vi "TLTSPB_Example.vi"() -> ()   [LabVIEW 2023]
uses:
  Program Files/National Instruments/LabVIEW 2020/instr.lib/TLTSP/TLTSP.llb/z_StateMachineVorlageV2011.ctl
panel:
  out "XY Graph":T1(graph)
  out "Humidity":dbl
  out "Temperature":dbl caption="Temperature Ch1"
  in  "Stop":bool
  in  "Start":bool
  in  "Quit":bool
  in  "Tab Control":enum32{"Page 1", "Page 2"}(tab)
  in  "error in":errorcluster
  out "error out":errorcluster
  in  "Handle":refnum<visa-resource-name>
  in  "State210":T2 caption="States"
  out "State100":T2 caption="States"
  out "user event out":refnum<user-event>
  out "Connected":bool
  out "UserEventRefNum":refnum<event-registration>
  out "Temperature 2":dbl[](array[numeric])
  out "Humidity 2":dbl[](array[numeric])
  out "Time":timestamp[](array[timestamp])
  in  "Delay [ms]":u32=50
  out "Serial Number":string
  out "Device Name":string
  out "Manufacturer Name":string
  out "Firmware Revision":string
  out "Statuszeile":string
  # "Thorlabs TSP01B Example"
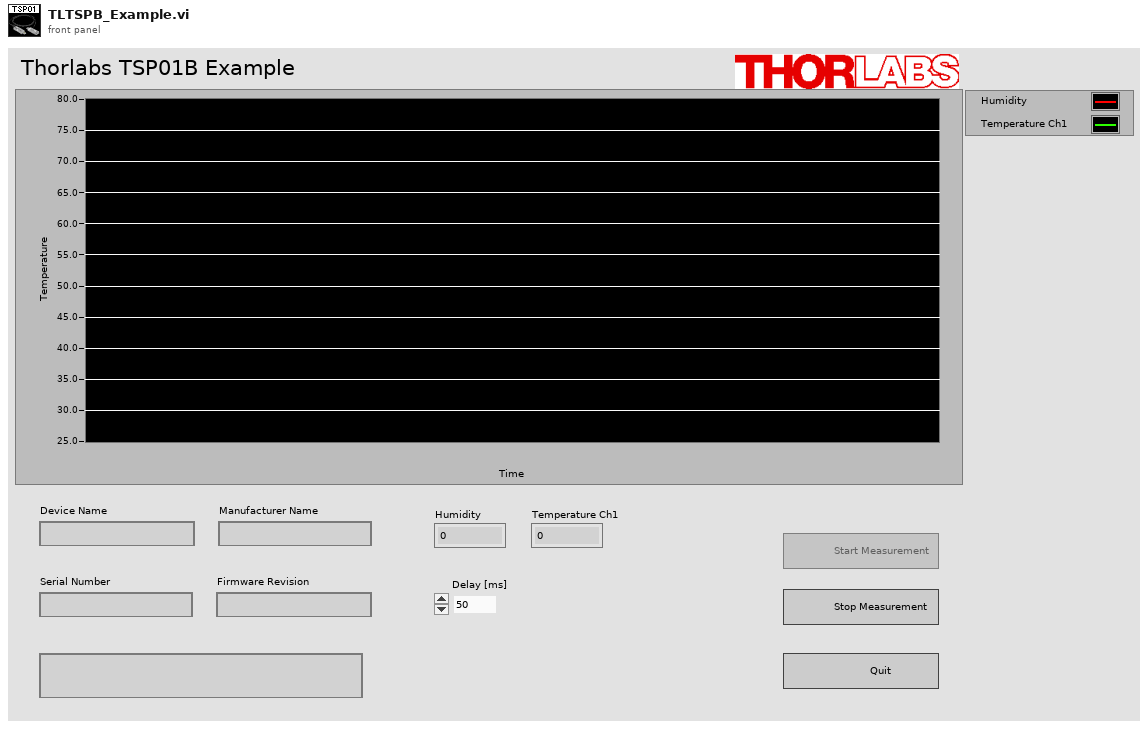
[diagram p1: front panel]
types:
  T1 = cluster{"Time":timestamp[], "Temperature":dbl[]}[]
  T2 = typedef "z_StateMachineVorlageV2011.ctl" = enum16{"Initialize", "1", "2", "3", "4", "5", "6", "7", "8", "9", "10", "15", "20", "25", "30", "35", "40", "45", "50", "55", "59", "60", "65", "70", "75", "76", "77", "78", "79", "80", "85", "90", "91", "92", "93", "94", "95", "96", "97", "98", "99", "100", "105", "110", "120", "130", "140", "150", "160", "170", "180", "190", "200", "205", "210", "215", "220", "230", "240", "245", "250", "255", "260", "270", "280", "290", "300", "310", "313", "315", "318", "320", "330", "340", "350", "360", "370", "380", "390", "400", "410", "420", "430", "440", "450", "460", "470", "480", "490", "500", "510", "520", "523", "525", "528", "530", "540", "550", "560", "570", "580", "590", "600", "605", "610", "620", "630", "640", "650", "660", "670", "680", "690", "700", "710", "720", "730", "740", "750", "760", "770", "780", "790", "800", "810", "820", "830", "840", "850", "860", "870", "880", "890", "900", "910", "920", "930", "940", "950", "960", "970", "980", "990", "1000", "1010", "1020", "1030", "1040", "1050", "1060", "1070", "1080", "1090", "1100", "1110", "1120", "1130", "1140", "1150", "1160", "1170", "1180", "1190", "1200", "1210", "1220", "1230", "1240", "1250", "1260", "1270", "1280", "1290", "1300", "1310", "1320", "1330", "1340", "1350", "1360", "1370", "1380", "1390", "1400", "1410", "1420", "1430", "1440", "1450", "1460", "1470", "1480", "1490", "1500", "Fehler I", "Fehler II", "Fehler III", "Fehler IV", "Fehler V", "Fehler VI", "Fehler VII", "Fehler VIII", "Fehler IX", "Fehler X", "Stop"}
  T3 = enum8{"Enabled", "Disabled", "Disabled and Grayed Out"}
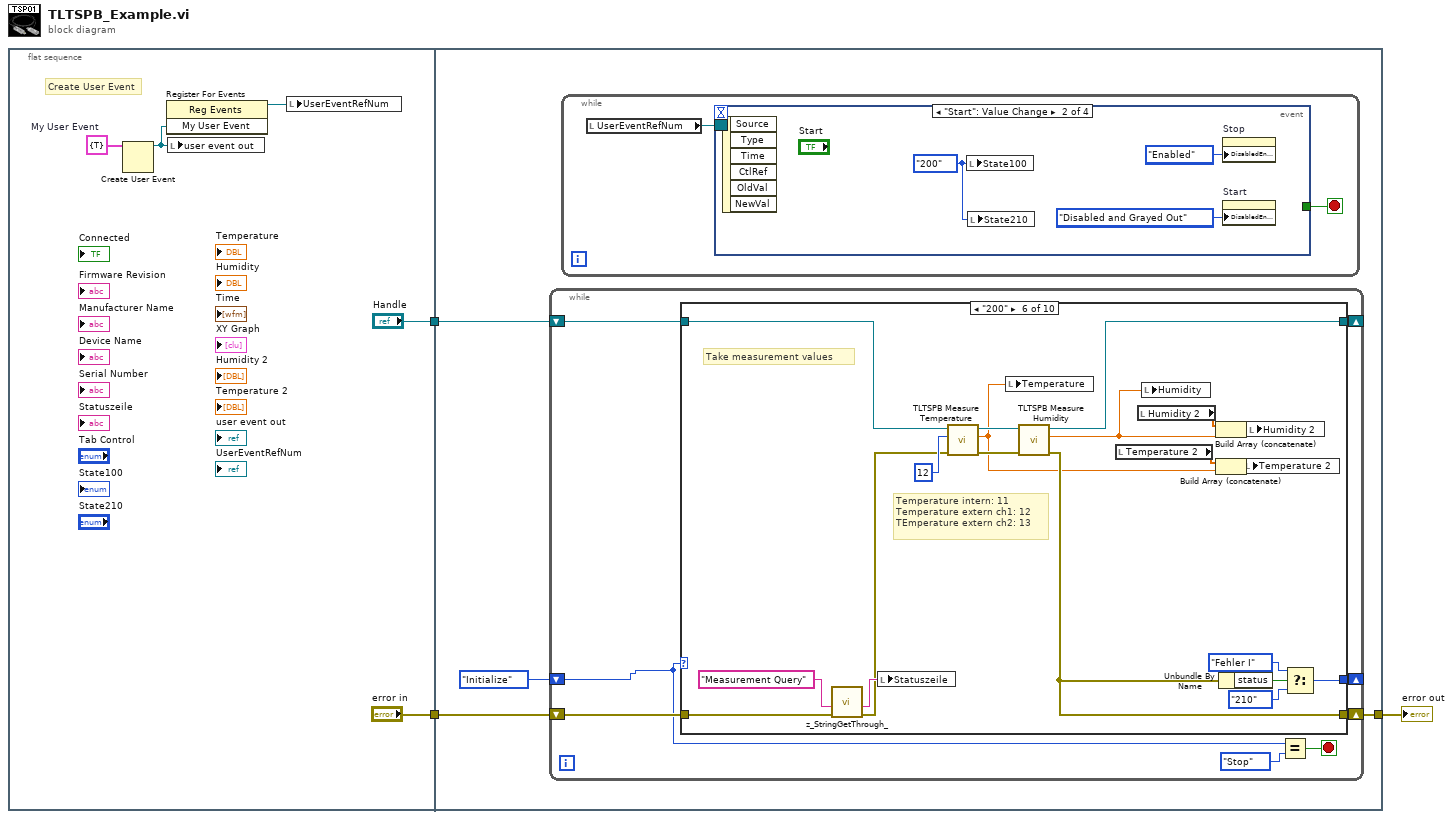
[diagram p0: block diagram]
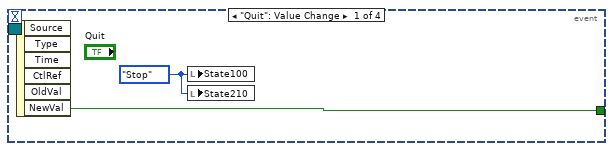
[diagram p2: hidden frame]
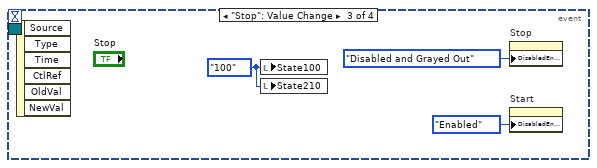
[diagram p3: hidden frame]
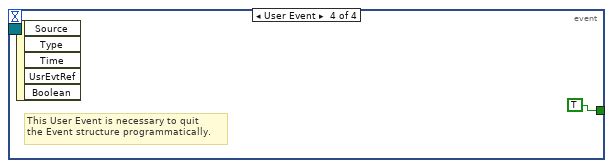
[diagram p4: hidden frame]
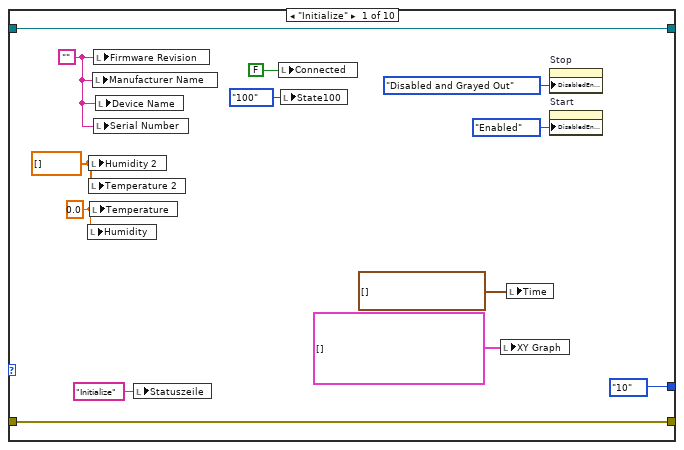
[diagram p5: hidden frame]
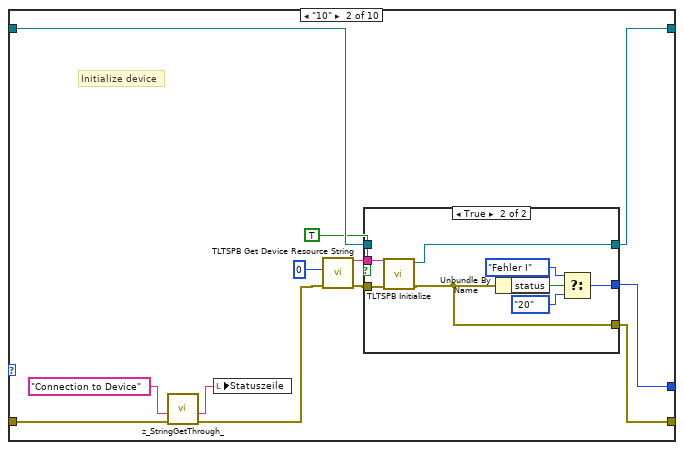
[diagram p6: hidden frame]
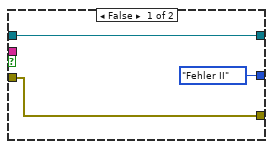
[diagram p7: hidden frame]
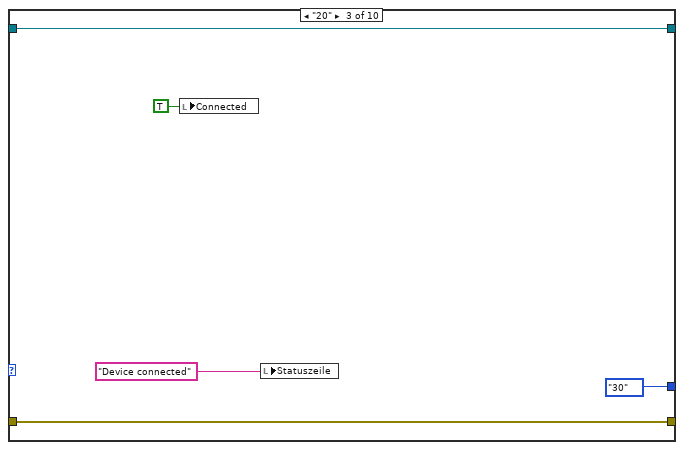
[diagram p8: hidden frame]
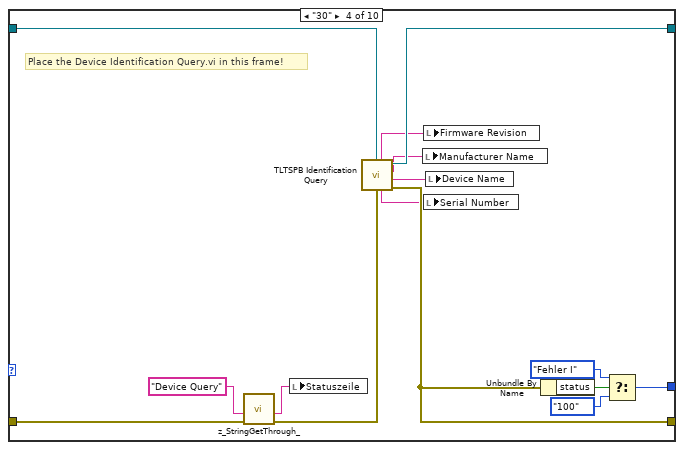
[diagram p9: hidden frame]
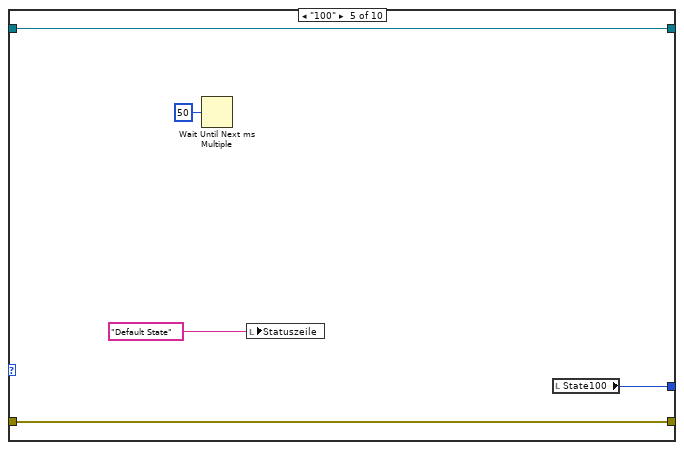
[diagram p10: hidden frame]
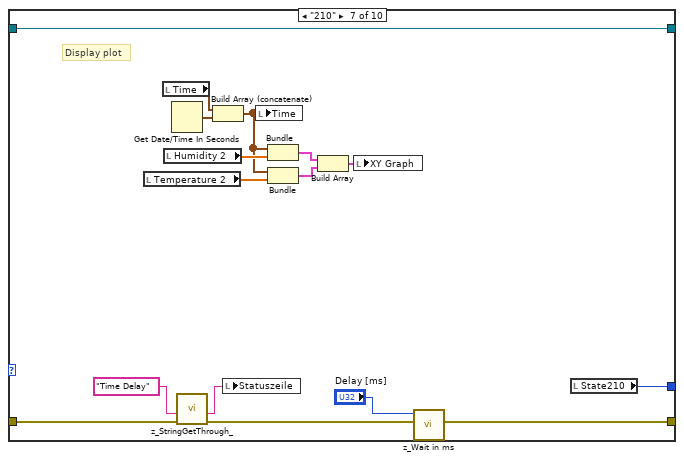
[diagram p11: hidden frame]
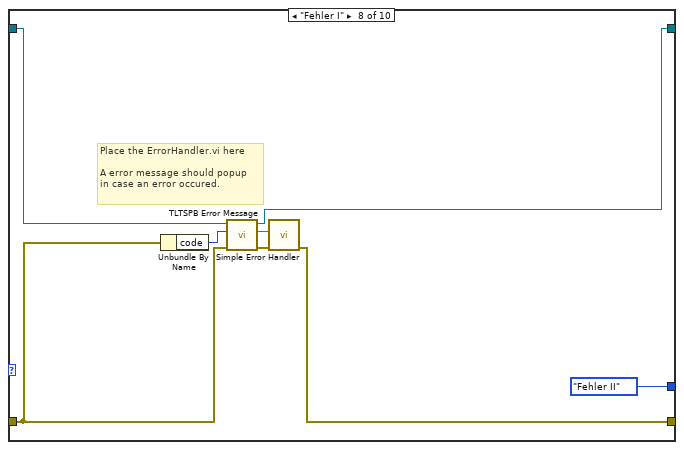
[diagram p12: hidden frame]
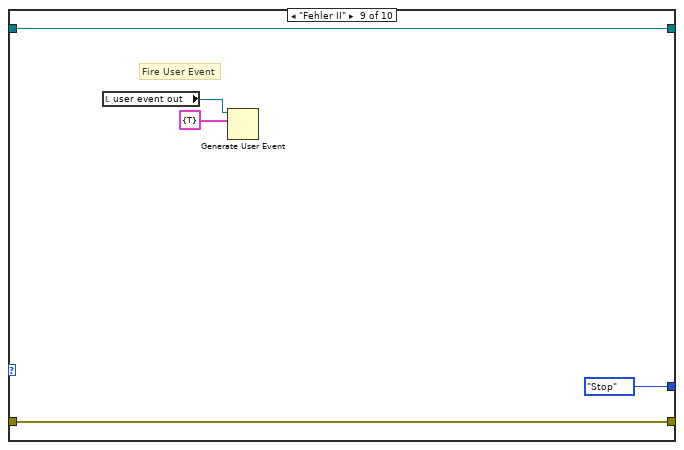
[diagram p13: hidden frame]
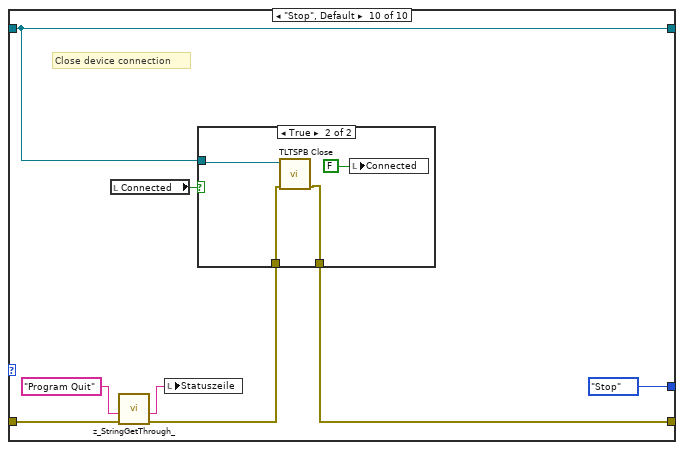
[diagram p14: hidden frame]
diagram:
  n1 = flat-sequence {
    tunnel: ["error in"] -> w3
    tunnel: ["Handle"] -> w1
    tunnel: w3 -> [w11]
    tunnel: [w10] -> w2
    tunnel: w1 -> [w9]
    frame #0 {
      w7 = cluster{"Boolean":bool} {"Boolean"=TRUE}  # My User Event
      # "Create User Event"
      n2 = Create User Event(user event datatype=w7) -> (user event=w8:refnum<user-event>)  [unwired: 1 in, 1 out]
      n3 = register-events(w8) -> (reference out=w6:refnum<event-registration>)  [unwired: 2 in, 1 out]
      n4 = local write "user event out"(w8) -> ()
      n5 = local write "UserEventRefNum"(w6) -> ()
    }
    frame #1 {
      n6 = while {
        shift-right: [w31] -> _
        shift-left: z_StateMachineVorlageV2011."Initialize" ("States") -> [w24]
        shift-right: [w27] -> w10
        shift-left: w11 -> [w28]
        shift-right: [w25] -> _
        shift-left: w9 -> [w26]
        stop <- w29 stop-if-true
        n7 = case shown="\"200\"" w24 {
          tunnel: [z_StateMachineVorlageV2011."10" ("States") w56 z_StateMachineVorlageV2011."30" ("States") w84 w92 w109 w127 z_StateMachineVorlageV2011."Fehler II" ("States") z_StateMachineVorlageV2011."Stop" ("States") z_StateMachineVorlageV2011."Stop" ("States")] -> w31
          tunnel: w28 -> [w40 w52 w70 w81 w89 w106 w124 w133 w137 w144]
          tunnel: [w40 w55 w70 w77 w89 w96 w121 w129 w137 w142] -> w27
          tunnel: w26 -> [w39 w54 w69 w80 w90 w94 w128 w134 w138 w147]
          tunnel: [w39 w53 w69 w78 w90 w97 w128 w135 w138 w147] -> w25
          frame "Initialize" {
            w32 = 0.0 ("Temperature")
            w35 = dbl[] [] ("Humidity")
            w41 = ""
            n8 = local write "Humidity"(w32) -> ()
            n9 = local write "Humidity 2"(w35) -> ()
            n10 = local write "Temperature 2"(w35) -> ()
            n11 = local write "Temperature"(w32) -> ()
            n12 = local write "Manufacturer Name"(w41) -> ()
            n13 = local write "Firmware Revision"(w41) -> ()
            n14 = local write "Serial Number"(w41) -> ()
            n15 = local write "Device Name"(w41) -> ()
            n16 = local write "Statuszeile"("Initialize" ("Statuszeile")) -> ()
            n17 = local write "Connected"(FALSE ("Quit")) -> ()
            n18 = local write "State100"(z_StateMachineVorlageV2011."100" ("State100")) -> ()
            n19 = local write "XY Graph"(T1 [] ("XY Graph")) -> ()
            n20 = local write "Time"(timestamp[] [] ("Time")) -> ()
            n21 = property on="Stop" class="Bool"("DisabledEnum"=T3."Disabled and Grayed Out" ("Disabled")) -> ()  [unwired: 2 in, 2 out]
            n22 = property on="Start" class="Bool"("DisabledEnum"=T3."Enabled" ("Disabled")) -> ()  [unwired: 2 in, 2 out]
          }
          frame "10" {
            # "Initialize device"
            n23 = call "z_StringGetThrough_.vi"("Error In"=w52, "String In"="Connection to Device") -> ("Error Out"=w49:errorcluster, "String Out"=w51:string)  [unwired: 8 in]
            n24 = local write "Statuszeile"(w51) -> ()
            n25 = call "TLTSPB Get Device Resource String.vi"("error in (no error)"=w49, "Device Index"=u32 0) -> ("error out"=w48:errorcluster, "Resource Name"=w47:string)  [unwired: 7 in, 1 out]
            n26 = case shown="True" TRUE {
              tunnel: w48 -> [w58 w63]
              tunnel: [z_StateMachineVorlageV2011."Fehler II" ("f") w64] -> w56
              tunnel: [w58 w62] -> w55
              tunnel: [w59 w61] -> w53
              tunnel: w54 -> [w59 _]
              tunnel: w47 -> [_ w60]
              frame False {
              }
              frame True {
                n27 = call "TLTSPB Initialize.vi"("error in (no error)"=w63, "resource name"=w60) -> ("error out"=w62:errorcluster, "instrument handle out"=w61:refnum<visa-resource-name>)  [unwired: 8 in]
                n28 = Unbundle By Name(w62) -> ("status"=w65:bool)
                n29 = Select(t=z_StateMachineVorlageV2011."Fehler I" ("States"), s=w65, f=z_StateMachineVorlageV2011."20") -> (s? t:f=w64:T2)
              }
            }
          }
          frame "20" {
            n30 = local write "Connected"(TRUE ("Connected")) -> ()
            n31 = local write "Statuszeile"("Device connected" ("String In")) -> ()
          }
          frame "30" {
            # "Place the Device Identification Query.vi in this frame!"
            n32 = call "z_StringGetThrough_.vi"("Error In"=w81, "String In"="Device Query") -> ("Error Out"=w79:errorcluster, "String Out"=w83:string)  [unwired: 8 in]
            n33 = local write "Statuszeile"(w83) -> ()
            n34 = call "TLTSPB Identification Query.vi"("error in (no error)"=w79, "instrument handle"=w80) -> ("error out"=w77:errorcluster, "Device Name"=w75:string, "Manufacturer Name"=w74:string, "instrument handle out"=w78:refnum<visa-resource-name>, "Serial Number"=w76:string, "Firmware Revision"=w73:string)  [unwired: 4 in]
            n35 = local write "Manufacturer Name"(w74) -> ()
            n36 = local write "Firmware Revision"(w73) -> ()
            n37 = local write "Serial Number"(w76) -> ()
            n38 = local write "Device Name"(w75) -> ()
            n39 = Unbundle By Name(w77) -> ("status"=w85:bool)
            n40 = Select(t=z_StateMachineVorlageV2011."Fehler I" ("States"), s=w85, f=z_StateMachineVorlageV2011."100") -> (s? t:f=w84:T2)
          }
          frame "100" {
            n41 = Wait Until Next ms Multiple(millisecond multiple=u32 50) -> ()  [unwired: 1 out]
            n42 = local write "Statuszeile"("Default State" ("String In")) -> ()
            n43 = local read "State100"() -> (w92:T2)
          }
          frame "200" {
            # "Temperature intern: 11\nTemperature extern ch1: 12\nTEmperature extern ch2: 13"
            # "Take measurement values"
            n44 = call "z_StringGetThrough_.vi"("Error In"=w106, "String In"="Measurement Query") -> ("Error Out"=w93:errorcluster, "String Out"=w108:string)  [unwired: 8 in]
            n45 = local write "Statuszeile"(w108) -> ()
            n46 = call "TLTSPB Measure Temperature.vi"("error in (no error)"=w93, "Channel (Temperatur Channel 1)"=u16 12 ("Channel (1)"), "instrument handle"=w94) -> ("error out"=w99:errorcluster, "Temperature"=w95:dbl, "instrument handle out"=w100:refnum<visa-resource-name>)  [unwired: 6 in]
            n47 = local write "Temperature"(w95) -> ()
            n48 = call "TLTSPB Measure Humidity.vi"("error in (no error)"=w99, "instrument handle"=w100) -> ("error out"=w96:errorcluster, "Humidity"=w98:dbl, "instrument handle out"=w97:refnum<visa-resource-name>)  [unwired: 7 in]
            n49 = local read "Temperature 2"() -> (w103:dbl[])
            n50 = local read "Humidity 2"() -> (w102:dbl[])
            n51 = local write "Humidity"(w98) -> ()
            n52 = Build Array (concatenate)(w102, w98) -> (w104:dbl[])
            n53 = Build Array (concatenate)(w103, w95) -> (w105:dbl[])
            n54 = Unbundle By Name(w96) -> ("status"=w110:bool)
            n55 = local write "Temperature 2"(w105) -> ()
            n56 = local write "Humidity 2"(w104) -> ()
            n57 = Select(t=z_StateMachineVorlageV2011."Fehler I" ("States"), s=w110, f=z_StateMachineVorlageV2011."210") -> (s? t:f=w109:T2)
          }
          frame "210" {
            # "Display plot"
            n58 = local read "Temperature 2"() -> (w119:dbl[])
            n59 = local read "Time"() -> (w115:timestamp[])
            n60 = local read "Humidity 2"() -> (w120:dbl[])
            n61 = Get Date/Time In Seconds() -> (seconds since 1Jan1904=w114:timestamp)
            n62 = call "z_StringGetThrough_.vi"("Error In"=w124, "String In"="Time Delay") -> ("Error Out"=w123:errorcluster, "String Out"=w126:string)  [unwired: 8 in]
            n63 = Build Array (concatenate)(w115, w114) -> (w113:timestamp[])
            n64 = local write "Statuszeile"(w126) -> ()
            n65 = local write "Time"(w113) -> ()
            n66 = Bundle(w113, "Humidity 2"=w120) -> (w118:cluster{timestamp[], "Humidity 2":dbl[]})  [unwired: 1 in]
            n67 = Bundle(w113, "Temperature 2"=w119) -> (w117:cluster{timestamp[], "Temperature 2":dbl[]})  [unwired: 1 in]
            n68 = Build Array(w118, w117) -> (w116:cluster{timestamp[], "Temperature 2":dbl[]}[])
            n69 = local write "XY Graph"(w116) -> ()
            n70 = call "z_Wait in ms.vi"("Error In"=w123, "milliseconds to wait"="Delay [ms]") -> ("Error Out"=w121:errorcluster)  [unwired: 8 in, 1 out]
            n71 = local read "State210"() -> (w127:T2)
          }
          frame "Fehler I" {
            # "Place the ErrorHandler.vi here\n\nA error message should popup\nin case an error occured."
            n72 = Unbundle By Name(w133) -> ("code"=w132:i32)
            n73 = call "TLTSPB Error Message.vi"("error in (no error)"=w133, "Error Code (0)"=w132, "instrument handle"=w134) -> ("error out"=w130:errorcluster, "Error Message"=w131:string, "instrument handle out"=w135:refnum<visa-resource-name>)  [unwired: 6 in]
            n74 = call <vilib>:"Simple Error Handler.vi"("error source (\" \")"=w131, "error in (no error)"=w130) -> ("error out"=w129:errorcluster)  [unwired: 3 in, 4 out]
          }
          frame "Fehler II" {
            # "Fire User Event"
            n75 = local read "user event out"() -> (w140:refnum<user-event>)
            n76 = Generate User Event(user event=w140, event data cluster=cluster{"Boolean":bool} {"Boolean"=TRUE} ("event data")) -> ()  [unwired: 2 in, 2 out]
          }
          frame "Stop", Default {
            # "Close device connection"
            n77 = local read "Connected"() -> (w148:bool)
            n78 = call "z_StringGetThrough_.vi"("Error In"=w144, "String In"="Program Quit") -> ("Error Out"=w143:errorcluster, "String Out"=w146:string)  [unwired: 8 in]
            n79 = local write "Statuszeile"(w146) -> ()
            n80 = case shown="True" w148 {
              tunnel: w147 -> [_ w152]
              tunnel: w143 -> [w150 w153]
              tunnel: [w150 w151] -> w142
              frame False {
              }
              frame True {
                n81 = call "TLTSPB Close.vi"("error in (no error)"=w153, "instrument handle"=w152) -> ("error out"=w151:errorcluster)  [unwired: 9 in]
                n82 = local write "Connected"(FALSE ("Connected")) -> ()
              }
            }
          }
        }
        n83 = Equal?(x=w24, y=z_StateMachineVorlageV2011."Stop" ("States")) -> (x = y?=w29:bool)
      }
      n84 = while {
        stop <- w14 stop-if-true
        n85 = local read "UserEventRefNum"() -> (w13:refnum<event-registration>)
        n86 = event shown="[1] \"Start\": Value Change" {
          selector: w13 -> [_ _ _ _]
          dyn-events: _ -> [_ _ _ _]
          timeout: _ -> [_ _ _ _]
          tunnel: [w16 _ _ TRUE ("NewVal")] -> w14
          event "Quit": Value Change {
            w15 = z_StateMachineVorlageV2011."Stop" ("State100")
            n87 = event-data() -> ("NewVal"=w16:bool)  [unwired: 6 out]
            n88 = local write "State100"(w15) -> ()
            n89 = local write "State210"(w15) -> ()
          }
          event "Start": Value Change {
            (unwired) T3."Disabled and Grayed Out" ("Disabled")
            (unwired) T3."Enabled" ("Disabled")
            w18 = z_StateMachineVorlageV2011."200" ("State100")
            n90 = event-data() -> ()  [unwired: 7 out]
            n91 = local write "State100"(w18) -> ()
            n92 = local write "State210"(w18) -> ()
            n93 = property on="Stop" class="Bool"("DisabledEnum"=T3."Enabled" ("Disabled")) -> ()  [unwired: 2 in, 2 out]
            n94 = property on="Start" class="Bool"("DisabledEnum"=T3."Disabled and Grayed Out" ("Disabled")) -> ()  [unwired: 2 in, 2 out]
          }
          event "Stop": Value Change {
            w21 = z_StateMachineVorlageV2011."100" ("State100")
            n95 = event-data() -> ()  [unwired: 7 out]
            n96 = local write "State100"(w21) -> ()
            n97 = local write "State210"(w21) -> ()
            n98 = property on="Stop" class="Bool"("DisabledEnum"=T3."Disabled and Grayed Out" ("Disabled")) -> ()  [unwired: 2 in, 2 out]
            n99 = property on="Start" class="Bool"("DisabledEnum"=T3."Enabled" ("Disabled")) -> ()  [unwired: 2 in, 2 out]
          }
          event User Event {
            # "This User Event is necessary to quit\nthe Event structure programmatically."
            n100 = event-data() -> ()  [unwired: 6 out]
          }
        }
      }
    }
  }
  "error out" <- w2
